vi "SIFS_Read_IO_States.vi"(0 "VISA Name In":refnum<visa-resource-name>, 2 "ID":string, 3 "error in":errorcluster) -> (1 "Home Bit":bool, 4 "Run Bit":bool, 5 "VISA Name Out":refnum<visa-resource-name>, 6 "Error":bool, 7 "Status Byte":bool[](array[boolean]), 8 "error out":errorcluster)   [LabVIEW 2018]
panel:
  out "StrStates":string
  # "Index"
  # "Moving Error"
  # "Holding Error"
  # "Moving"
  # "I/O#1"
  # "I/O#2"
  # "I/O#3"
  # "Over Temperature"
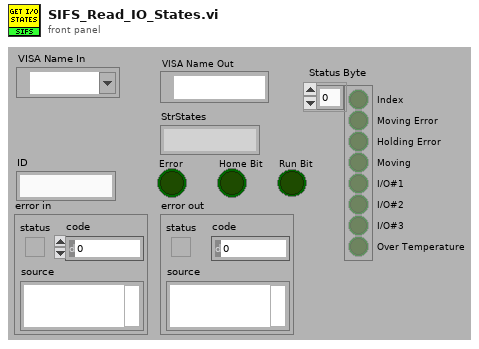
[diagram p1: front panel]
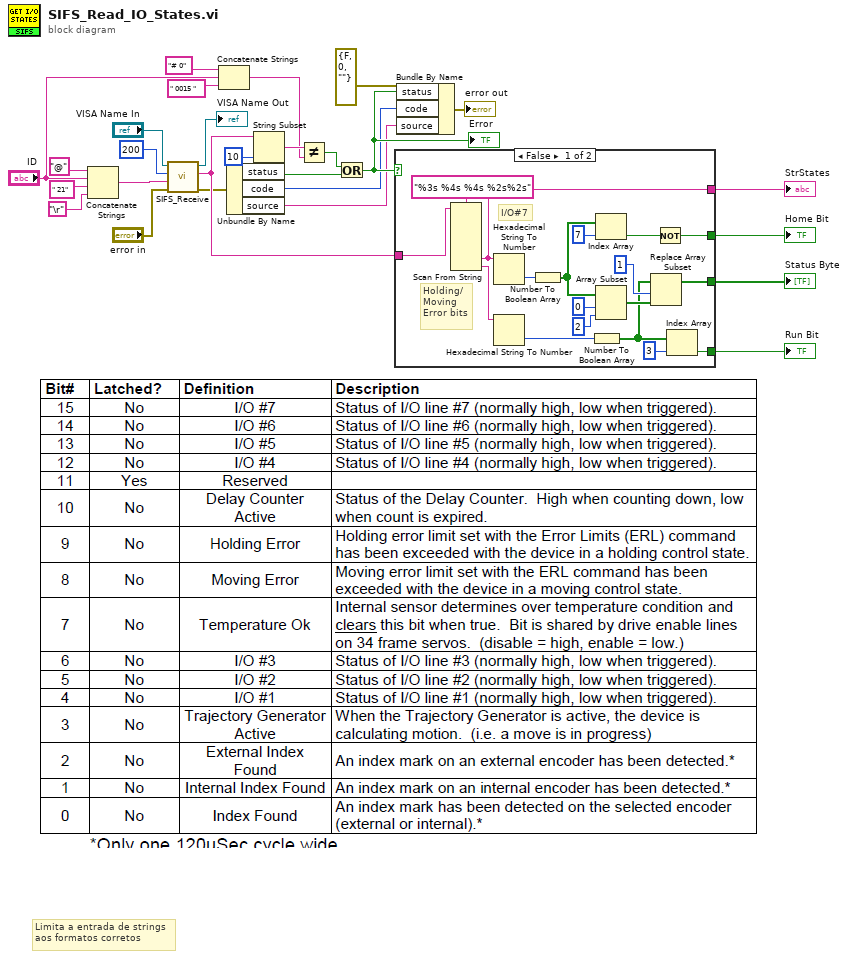
[diagram p0: block diagram]
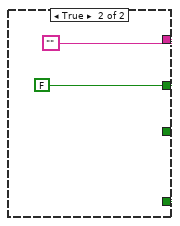
[diagram p2: hidden frame]
diagram:
  # "Limita a entrada de strings\naos formatos corretos"
  n1 = Concatenate Strings("@" ("string"), "ID", " 21", "\r") -> (w6:string)
  n2 = call "SIFS_Receive.vi"("error in"="error in", "Command to SIFS"=w6, "wait after tx"=u32 200 ("milliseconds to wait"), "VISA resource name"="VISA Name In") -> ("error out"=w1:errorcluster, "Response from SIFS"=w2:string, "VISA resource name out"=→"VISA Name Out":refnum<visa-resource-name>)  [unwired: 1 out]
  n3 = Concatenate Strings("# 0" ("string"), "ID", " 0015 ") -> (w20:string)
  n4 = Unbundle By Name(w1) -> ("status"=w17:bool, "code"=w9:i32, "source"=w8:string)
  n5 = String Subset(string=w2, length (rest)=10 ("length (rest)")) -> (substring=w25:string)  [unwired: 1 out]
  n6 = Not Equal?(x=w25, y=w20) -> (x != y?=w19:bool)
  n7 = Or(x=w19, y=w17) -> (x .or. y?=w12:bool)
  "Error" <- w12
  n8 = case shown="False" w12 {
    tunnel: w2 -> [w45 _]
    tunnel: [w43 ""] -> w16
    tunnel: [w28 w46] -> w15
    tunnel: [w33 _] -> w14
    tunnel: [w29 w46] -> w13
    frame False {
      # "Holding/\nMoving\nError bits"
      # "I/O#7"
      n9 = Scan From String(format string="%3s %4s %4s %2s%2s", input string=w45) -> (output 4=w43:string, output 5=w40:string)  [unwired: 2 in, 11 out]
      n10 = Hexadecimal String To Number(string=w43) -> (number=w42:u32)  [unwired: 3 out]
      n11 = Hexadecimal String To Number(string=w40) -> (number=w41:u32)  [unwired: 3 out]
      n12 = Number To Boolean Array(number=w42) -> (Boolean array=w37:bool[])
      n13 = Number To Boolean Array(number=w41) -> (Boolean array=w30:bool[])
      n14 = Index Array(array=w37, index=7) -> (element=w39:bool)
      n15 = Array Subset(array=w37, index=0, length=2) -> (w31:bool[])
      n16 = Replace Array Subset(array=w30, new element=w31, index=1) -> (w33:bool[])
      n17 = Not(x=w39) -> (.not. x?=w28:bool)
      n18 = Index Array(array=w30, index=3) -> (element=w29:bool)
    }
    frame True {
      w46 = FALSE
    }
  }
  "StrStates" <- w16
  "Status Byte" <- w14
  "Home Bit" <- w15
  "Run Bit" <- w13
  n19 = Bundle By Name(cluster=errorcluster {"status"=FALSE, "code"=0, "source"=""} ("error in"), "status"=w12, "code"=w9, "source"=w8) -> (→"error out":errorcluster)
